vi "iRobot UART Close.vi"(8 "error in":errorcluster, 11 "UART port in":T1) -> (0 "error out":errorcluster)   [LabVIEW 2010]
doc: "Closes the UART port connected to iRobot. The port must be reinitialized before reuse."
uses:
  UART Port Type.ctl
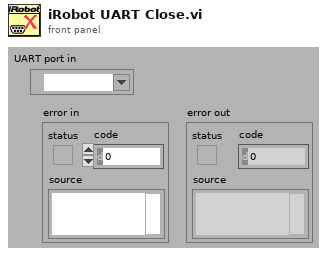
[diagram p1: front panel]
types:
  T1 = typedef "UART Port Type.ctl" = refnum<visa-resource-name>
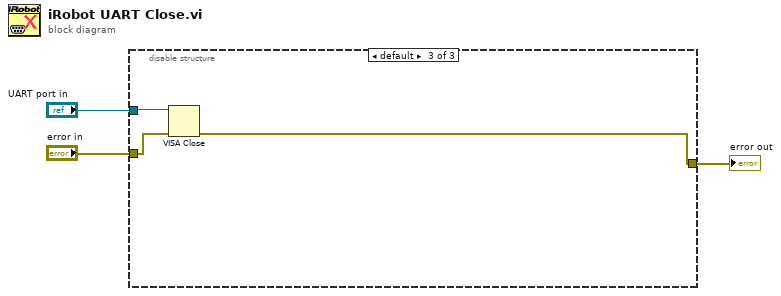
[diagram p0: block diagram]
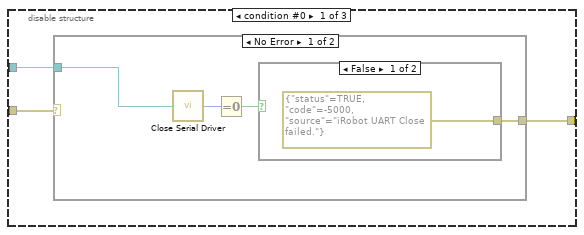
[diagram p2: hidden frame]
diagram:
  n1 = disable-structure shown="default" {
    disable-tunnel: "error in" -> [w6 _ w14]
    disable-tunnel: [w5 _ w13] -> w2
    disable-tunnel: "UART port in" -> [w4 _ w15]
    frame condition #0 {
      n2 = case shown="No Error" w6 {
        selector: w6 -> [_ w12]
        tunnel: [w8 w12] -> w5
        tunnel: w4 -> [w7 _]
        frame No Error {
          n3 = call <vilib>:"Close Serial Driver.vi"("port number"=w7) -> ("error"=w10:i32)
          n4 = Equal To 0?(x=w10) -> (x = 0?=w9:bool)
          n5 = case shown="False" w9 {
            tunnel: [errorcluster {"status"=TRUE, "code"=-5000, "source"="iRobot UART Close failed."} ("error out") _] -> w8
            frame False {
            }
            frame True {
              # "No error"
            }
          }
        }
        frame Error {
        }
      }
    }
    frame condition #1 {
      # "To be deployed..."
    }
    frame condition #2 (active) {
      n6 = VISA Close(VISA resource name=w15, error in (no error)=w14) -> (error out=w13:errorcluster)
    }
  }
  "error out" <- w2
